vi "Set Sparse Marker Indexes [SM] Core.vi"(8 "error in (no error)":errorcluster, 9 "Indexes Array":i64[](array[numeric]) caption="indexes array", 10 "Marker Name (\"\")":string caption="marker name (\"\")", 11 "CS++Fgen in":refnum<class "CS++Fgen.lvclass">) -> (0 "error out":errorcluster, 3 "CS++Fgen out":refnum<class "CS++Fgen.lvclass">)   [LabVIEW 2013, in "CS++Fgen.lvlib" / "CS++Fgen.lvclass"]
doc: "The VI sets the indexes associated with the sparse marker. These indexes may be coerced by the driver. Use the IviFgen Get Sparse Marker Indexes [SM] VI to find the coerced values.\n\nNote:\n\n(1) This VI is part of the IviFgenSparseMarker [SM] extension group."
uses:
  CS++Fgen.lvclass
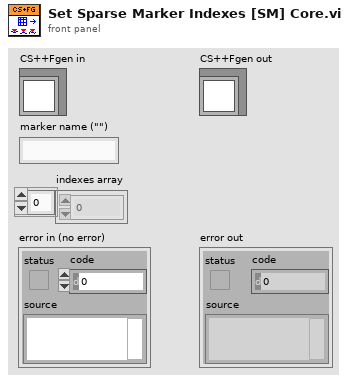
[diagram p1: front panel]
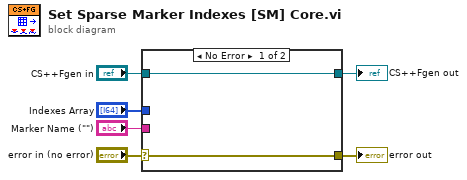
[diagram p0: block diagram]
diagram:
  n1 = case shown="No Error" "error in (no error)" {
    selector: "error in (no error)" -> [w7 w10]
    tunnel: [w7 w10] -> w5
    tunnel: [w8 w9] -> w3
    tunnel: "CS++Fgen in" -> [w8 w9]
    tunnel: "Marker Name (\"\")" -> [_ _]
    tunnel: "Indexes Array" -> [_ _]
    frame No Error {
    }
    frame Error {
    }
  }
  "error out" <- w5
  "CS++Fgen out" <- w3
